vi "spec_set_integration_time.vi"(8 "error in (no error)":errorcluster, 10 "integr time [s]":dbl, 11 "Qtegra in":refnum<class "Qtegra.lvclass">) -> (0 "error out":errorcluster, 2 "value out":string, 3 "Qtegra out":refnum<class "Qtegra.lvclass">)   [LabVIEW 2017, in "Qtegra.lvclass"]
doc: "sets the integration time of the spectrometer"
uses:
  Qtegra.lvclass
  \\Mac\Home/my data/University/Lamont/Software/LabView/MSControlSuite_Code/MSControl/Classes/Instrument/instrument.lvclass
  global variables.vi
  instrument.lvclass
  StatusLog/StatusLog.lvclass
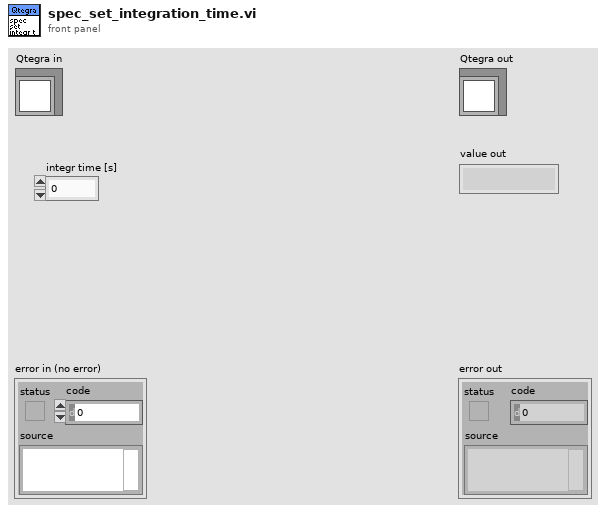
[diagram p1: front panel]
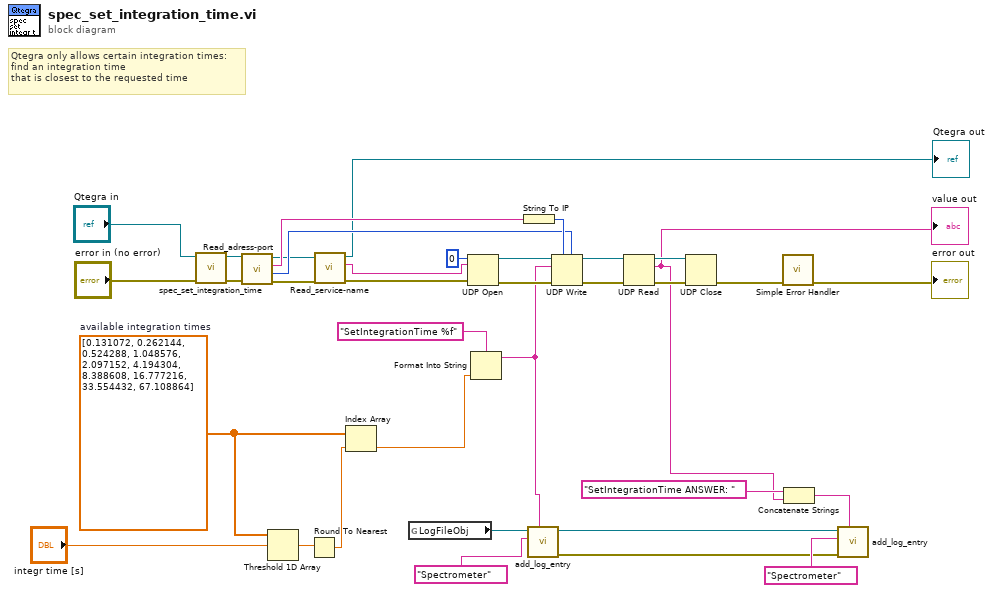
[diagram p0: block diagram]
diagram:
  w12 = dbl[] [0.131072, 0.262144, 0.524288, 1.048576, 2.097152, 4.194304, 8.388608, 16.777216, 33.554432, 67.108864]  # available integration times
  # "Qtegra only allows certain integration times:\nfind an integration time\nthat is closest to the requested time"
  n1 = call-parent "spec_set_integration_time.vi"("error in (no error)"="error in (no error)", "instrument in"="Qtegra in") -> ("error out"=w17:errorcluster, "instrument out"=w16:refnum<class "Qtegra.lvclass">)  [unwired: 7 in, 1 out]
  n2 = call "Read_adress-port.vi"("error in (no error)"=w17, "instrument in"=w16) -> ("error out"=w26:errorcluster, "port number"=w27:i32, "adress"=w34:string, "instrument out"=w25:refnum<class "Qtegra.lvclass">)  [unwired: 6 in]
  n3 = Threshold 1D Array(2:"integr time [s]", 3:w12) -> (0:w13:dbl)  [unwired: 1 in]
  n4 = Round To Nearest(number=w13) -> (nearest integer value=w11:dbl)
  n5 = call-dynamic "Read_service-name.vi"("error in (no error)"=w26, "instrument in"=w25) -> ("error out"=w24:errorcluster, "service name"=w23:string, "instrument out"=→"Qtegra out":refnum<class "Qtegra.lvclass">)  [unwired: 7 in]
  n6 = Index Array(array=w12, index=w11) -> (element=w10:dbl)
  n7 = global read "global variables.vi" "LogFileObj"() -> (w7:refnum<class "StatusLog.lvclass">)
  n8 = UDP Open(8:w24, 10:w23, 11:u16 0 ("port")) -> (port=w30:refnum<k16>, 0:w31:errorcluster)  [unwired: 2 in, 1 out]
  n9 = Format Into String(format string="SetIntegrationTime %f", w10) -> (resulting string=w2:string)  [unwired: 2 in, 1 out]
  n10 = String To IP(1:w34) -> (0:w33:u32)
  n11 = call-dynamic "add_log_entry.vi"("new entry"=w2, "log identifiers"="Spectrometer", "StatusLog in"=w7) -> ("error out"=w3:errorcluster, "StatusLog out"=w6:refnum<class "StatusLog.lvclass">)  [unwired: 5 in]
  n12 = UDP Write(address=w33, port or service name=w27, connection ID=w30, data in=w2, 8:w31) -> (error out=w28:errorcluster, 3:w29:refnum<k16>)  [unwired: 1 in]
  n13 = UDP Read(connection ID=w29, 8:w28) -> (data out=w1:string, error out=w21:errorcluster, 3:w19:refnum<k16>)  [unwired: 2 in, 2 out]
  "value out" <- w1
  n14 = UDP Close(connection ID=w19, 8:w21) -> (error out=w20:errorcluster)  [unwired: 1 out]
  n15 = call <vilib>:"Simple Error Handler.vi"("error in (no error)"=w20) -> ("error out"=→"error out":errorcluster)  [unwired: 4 in, 4 out]
  n16 = Concatenate Strings("SetIntegrationTime ANSWER: ", w1) -> (w4:string)
  n17 = call-dynamic "add_log_entry.vi"("new entry"=w4, "error in (no error)"=w3, "log identifiers"="Spectrometer", "StatusLog in"=w6) -> ()  [unwired: 4 in, 2 out]
